vi "Exponential Decay Fitting.vi"(0 "Time":dbl[](array[numeric]), 1 "Concentration":dbl[](array[numeric]), 2 "Valve Off Index":i32=47971, 3 "Peak Value":dbl) -> (7 "Exponential Fit":cluster{dbl[], "Best Exponential Fit":dbl[]}, 9 "Parameter Names":string[](array[string]), 10 "Parameter Values":dbl[](array[numeric]))   [LabVIEW 2022 SP3]
uses:
  <vilib>/Analysis/NI_AALPro.lvlib
  <vilib>/Analysis/6fits.llb/Curve Fitting Criteria.ctl
panel:
  out "Amplitude":dbl
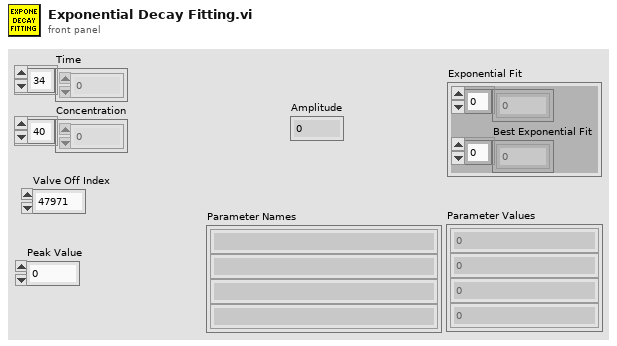
[diagram p1: front panel]
types:
  T1 = typedef "NI_AALPro.lvlib/Curve Fitting Criteria.ctl" = u16
  T2 = cluster{"amp min":dbl, "amp max":dbl, "damping min":dbl, "damping max":dbl, "offset min":dbl, "offset max":dbl}
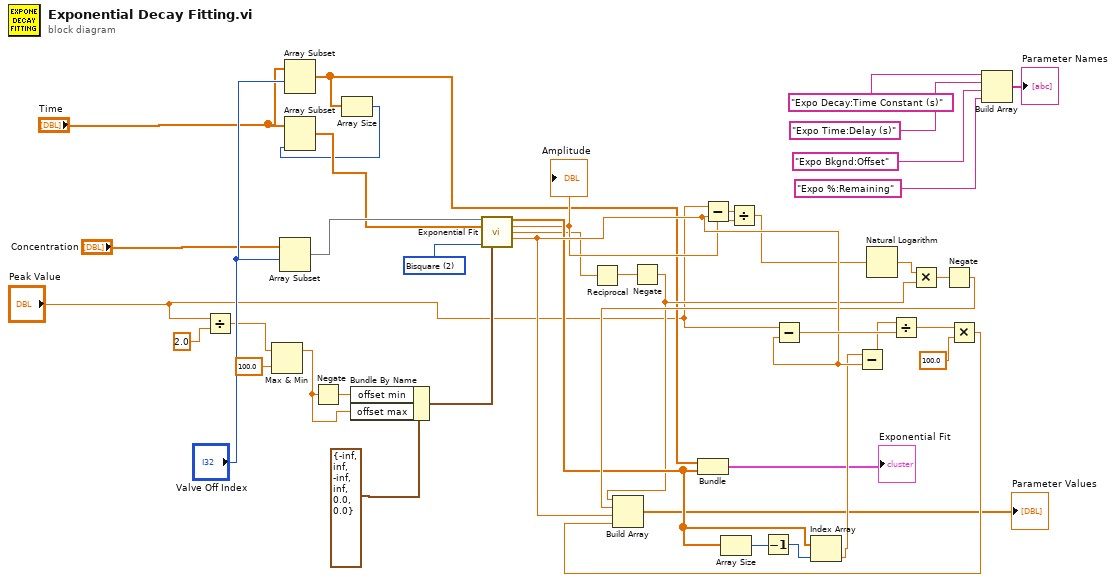
[diagram p0: block diagram]
diagram:
  w19 = T1 2 items=["Least Square", "Least Absolute Residual", "Bisquare"] ("method")
  n1 = Divide(x="Peak Value", y=2.0) -> (x/y=w14:dbl)
  n2 = Max & Min(x=w14, y=100.0) -> (max(x,y)=w17:dbl)  [unwired: 1 out]
  n3 = Array Subset(array="Concentration", index="Valve Off Index") -> (w39:dbl[])  [unwired: 1 in]
  n4 = Array Subset(array="Time", index="Valve Off Index") -> (w21:dbl[])  [unwired: 1 in]
  n5 = Negate(x=w17) -> (-x=w16:dbl)
  n6 = Array Size(array=w21) -> (size(s)=w22:i32)
  n7 = Array Subset(array="Time", length=w22) -> (w23:dbl[])  [unwired: 1 in]
  n8 = Bundle By Name(cluster=T2 {"amp min"=-inf, "amp max"=inf, "damping min"=-inf, "damping max"=inf, "offset min"=0.0, "offset max"=0.0} ("parameter bounds"), "offset min"=w16, "offset max"=w17) -> (w20:T2)
  n9 = call <vilib>:"Exponential Fit.vi"("Y"=w39, "X"=w23, "method"=w19, "parameter bounds"=w20) -> ("Best Exponential Fit"=w32:dbl[], "amplitude"=w25:dbl, "damping"=w10:dbl, "offset"=w41:dbl)  [unwired: 6 in, 2 out]
  "Amplitude" <- w25
  n10 = Reciprocal(x=w10) -> (1/x=w11:dbl)
  n11 = Negate(x=w11) -> (-x=w27:dbl)
  n12 = Bundle(w21, "Best Exponential Fit"=w32) -> (→"Exponential Fit":cluster{dbl[], "Best Exponential Fit":dbl[]})  [unwired: 1 in]
  n13 = Subtract(x="Peak Value", y=w41) -> (x-y=w24:dbl)
  n14 = Array Size(array=w32) -> (size(s)=w30:i32)
  n15 = Divide(x=w24, y=w25) -> (x/y=w29:dbl)
  n16 = Decrement(x=w30) -> (x-1=w31:i32)
  n17 = Subtract(x="Peak Value", y=w41) -> (x-y=w42:dbl)
  n18 = Index Array(array=w32, index=w31) -> (element=w33:dbl)
  n19 = Subtract(x=w33, y=w41) -> (x-y=w34:dbl)
  n20 = Natural Logarithm(1:w29) -> (0:w26:dbl)
  n21 = Divide(x=w34, y=w42) -> (x/y=w35:dbl)
  n22 = Multiply(x=w26, y=w27) -> (x*y=w28:dbl)
  n23 = Negate(x=w28) -> (-x=w37:dbl)
  n24 = Multiply(x=w35, y=100.0) -> (x*y=w40:dbl)
  n25 = Build Array(w27, w37, w41, w40) -> (→"Parameter Values":dbl[])
  n26 = Build Array("Expo Decay:Time Constant (s)", "Expo Time:Delay (s)", "Expo Bkgnd:Offset", "Expo %:Remaining") -> (→"Parameter Names":string[])
